vi "CANOpen_NMT_Main.vi"(6 "EM GB NG conf":T3(array[cluster])=[{"Emergency"={"Enable"=TRUE}, "Heartbeat and Node Guarding"={"Mode"=enum."None", "Guard Time (ms)"=5, "Consumer Time (ms)"=5}}, {"Emergency"={"Enable"=TRUE}, "Heartbeat and Node Guarding"={"Mode"=enum."None", "Guard Time (ms)"=5, "Consumer Time (ms)"=5}}], 7 "Period":i64=10, 8 "error in (no error)":errorcluster, 9 "stop in":bool, 10 "Nodes":T4[](array[typedef])=[{"RPDOs"=[], "TPDOs"=[], "Node ID"=1, "SDOs"=[], "Dynamic SDOs"=[], "NMT"={"Node run state"=0, "Emergency"=FALSE, "HB NG"={"Mode"=enum."NG", "Update Time"=128, "Static detect in None"=enum."HB"}, "Delay for opp. state (ms)"=5.0, "Node init static SDO state"=1, "Stop and Reset on Shutdown"=FALSE}}, {"RPDOs"=[], "TPDOs"=[], "Node ID"=2, "SDOs"=[], "Dynamic SDOs"=[], "NMT"={"Node run state"=0, "Emergency"=FALSE, "HB NG"={"Mode"=enum."NG", "Update Time"=128, "Static detect in None"=enum."HB"}, "Delay for opp. state (ms)"=5.0, "Node init static SDO state"=1, "Stop and Reset on Shutdown"=FALSE}}] {"NMT"."Node init static SDO state" items=["start remote node"=1, "enter pre-operational"=128]; "NMT"."Node run state" items=["start remote node"=1, "stop remote node"=2, "enter pre-operational"=128, "reset node"=129, "reset communication"=130]; "Dynamic SDOs"."Sub-Index (0)" format="%.0x"; "Dynamic SDOs"."Object Index" format="%.0x"; "Dynamic SDOs"."Block Data" format="%.0x"; "RPDOs"."PDO Channel" items=["PDO 1", "PDO 2", "PDO 3", "PDO 4"]; "RPDOs"."Parameters"."Bit Offset" max=8 step=1; "RPDOs"."Parameters"."Byte Offset" max=8 step=1; "TPDOs"."PDO Channel" items=["PDO 1", "PDO 2", "PDO 3", "PDO 4"]; "TPDOs"."Parameters"."Bit Offset" max=8 step=1; "TPDOs"."Parameters"."Byte Offset" max=8 step=1; "SDOs"."Sub-Index (0)" format="%.0x"; "SDOs"."Object Index" format="%.0x"; "SDOs"."Block Data" format="%.0x"}, 11 "interface object in":refnum<k20>) -> (0 "error out":errorcluster, 1 "Timestamp":timestamp, 2 "emergency message":T13 {"manufacturer specific error field" format="%.0x"; "error register" format="%.0x"; "error code" format="%.0x"}, 3 "interface object out":refnum<k20>, 5 "Is New?":bool)   [LabVIEW 2021, in "CANOpen Addon Engine.lvlib"]
uses:
  CANOpen Addon Engine.lvlib
  SubVIS/CANOpen_Node Message Settings.ctl
  Shared/CANOpen_PDO Settings.ctl
  Shared/CANOpen_PDO Parameter Settings.ctl
  Shared/CANOpen_PDO Data Type.ctl
  Shared/CANopen Byte Order.ctl
  Shared/CANOpen_SDO Settings.ctl
  SubVIS/CANOpen_NMT Settings.ctl
  Shared/CanOpen_NMT_Config.ctl
  Shared/CanOpen_NMT_Static detect.ctl
  Shared/CANOpen_Emergency Settings.ctl
  Shared/CANOpen_Heartbeat and Node Guarding Settings.ctl
  Emergency VI states.ctl
  <vilib>/Platform/TimedLoop/XDataNode/timing_clust.ctl
  <vilib>/Platform/TimedLoop/XDataNode/nitl_modes.ctl
  <vilib>/Platform/TimedLoop/XDataNode/wakeup.ctl
  <vilib>/CANopenLib/CANOPEN.llb/CANopen Emergency Create.vi
  <vilib>/CANopenLib/CANOPEN.llb/CANopen Emergency Start.vi
  <vilib>/CANopenLib/CANOPEN.llb/CANopen Emergency Read.vi
  <vilib>/CANopenLib/CANOPEN.llb/CANopen Emergency Close.vi
  <vilib>/Platform/TimedLoop/XDataNode/XDataNode.xnode
  <vilib>/Platform/TimedLoop/XDataNode/XDNodeRunTimeDep.lvlib
  Shared/CANOpen Addon Shared.lvlib
panel:
  # "LSB"
  # "MSB"
  # "LSB"
  # "MSB"
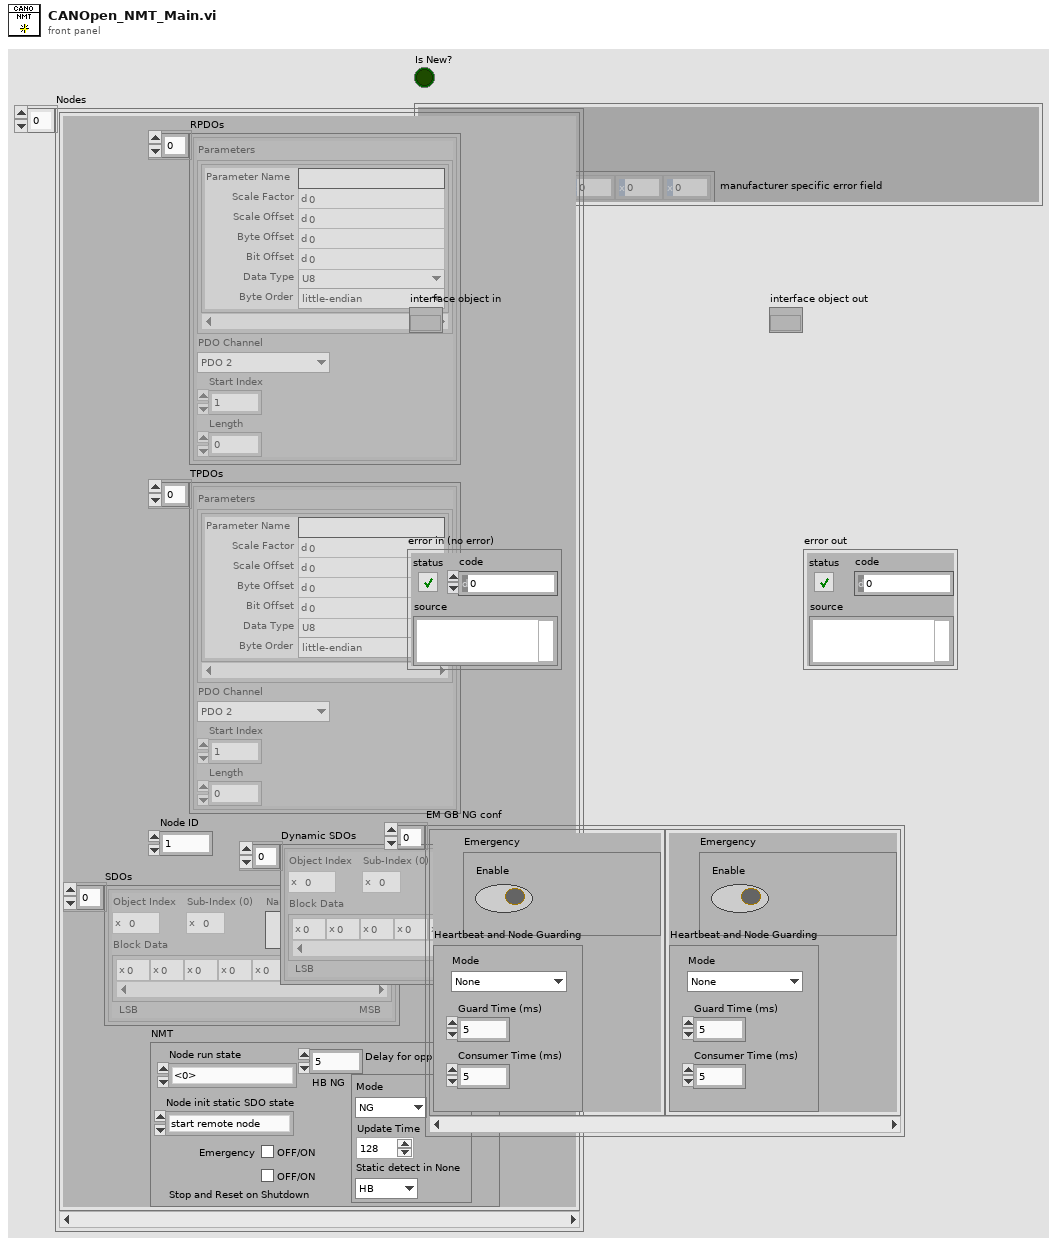
[diagram p1: front panel]
types:
  T1 = typedef "CANOpen Addon Shared.lvlib/CANOpen_Emergency Settings.ctl" = cluster{"Enable":bool}
  T2 = typedef "CANOpen Addon Shared.lvlib/CANOpen_Heartbeat and Node Guarding Settings.ctl" = cluster{"Mode":enum16{"None", "Hearbeat", "Node Guarding"}, "Guard Time (ms)":u16, "Consumer Time (ms)":u16}
  T3 = cluster{"Emergency":T1, "Heartbeat and Node Guarding":T2}[]
  T4 = typedef "CANOpen Addon Engine.lvlib/CANOpen_Node Message Settings.ctl" = cluster{"RPDOs":T5[], "TPDOs":T5[], "Node ID":u8, "SDOs":T9[], "Dynamic SDOs":T9[], "NMT":T10}
  T5 = typedef "CANOpen Addon Shared.lvlib/CANOpen_PDO Settings.ctl" = cluster{"Parameters":T6[], "PDO Channel":u8, "Start Index":u32, "Length":u32}
  T6 = typedef "CANOpen Addon Shared.lvlib/CANOpen_PDO Parameter Settings.ctl" = cluster{"Parameter Name":string, "Scale Factor":dbl, "Scale Offset":dbl, "Byte Offset":u8, "Bit Offset":u8, "Data Type":T7, "Byte Order":T8}
  T7 = typedef "CANOpen Addon Shared.lvlib/CANOpen_PDO Data Type.ctl" = enum16{"U8", "U16", "U32", "I8", "I16", "I32", "Single", "Double", "Boolean"}
  T8 = typedef "CANOpen Addon Shared.lvlib/CANopen Byte Order.ctl" = enum16{"big-endian network order", "little-endian"}
  T9 = typedef "CANOpen Addon Shared.lvlib/CANOpen_SDO Settings.ctl" = cluster{"Object Index":u16, "Sub-Index (0)":u8, "Block Data":u8[], "Name":string}
  T10 = typedef "CANOpen Addon Engine.lvlib/CANOpen_NMT Settings.ctl" = cluster{"Node run state":u16, "Emergency":bool, "HB NG":T11, "Delay for opp. state (ms)":dbl, "Node init static SDO state":u16, "Stop and Reset on Shutdown":bool}
  T11 = typedef "CANOpen Addon Shared.lvlib/CanOpen_NMT_Config.ctl" = cluster{"Mode":T12, "Update Time":u16, "Static detect in None":T12}
  T12 = typedef "CANOpen Addon Shared.lvlib/CanOpen_NMT_Static detect.ctl" = enum16{"None", "HB", "NG"}
  T13 = cluster{"error code":u16, "error register":u8, "manufacturer specific error field":u8[]}
  T14 = typedef "CANOpen Addon Engine.lvlib/Emergency VI states.ctl" = enum16{"Init", "Running ", "Shutdown"}
  T15 = typedef "XDNodeRunTimeDep.lvlib/timing_clust.ctl" = cluster{"Expected End [f-1]":u64, "Actual End [f-1]":u64, "Finished Late? [f-1]":bool, "Expected End [i-1]":u64, "Actual End [i-1]":u64, "Finished Late? [i-1]":bool, "Expected Start [i]":u64, "Actual Start [i]":u64, "Expected Start [f]":u64, "Actual Start [f]":u64, "Source Name":string, "Structure Name":string, "Period":i64, "Deadline":i64, "Offset":i64, "Start":i64, "Priority":i32, "Timeout":i32, "Mode":T16, "Wakeup Reason":T17, "Error":errorcluster, "Source Type":string, "Secondary Source Type":string, "Global End Time":u64, "Global Start Time":u64, "Frame Duration":u64, "Iteration Duration":u64, "Assigned CPU":i32, "I/O Scan Engine Mode":u32}
  T16 = typedef "XDNodeRunTimeDep.lvlib/nitl_modes.ctl" = enum32{"No Change", "Process missed periods, maintain original phase", "Discard missed periods, maintain original phase", "Process missed periods, ignore original phase", "Discard missed periods, ignore original phase"}
  T17 = typedef "XDNodeRunTimeDep.lvlib/wakeup.ctl" = enum32{"Normal", "Aborted", "Asynchronous wakeup", "Timing source error", "Timed loop error", "Timeout"}
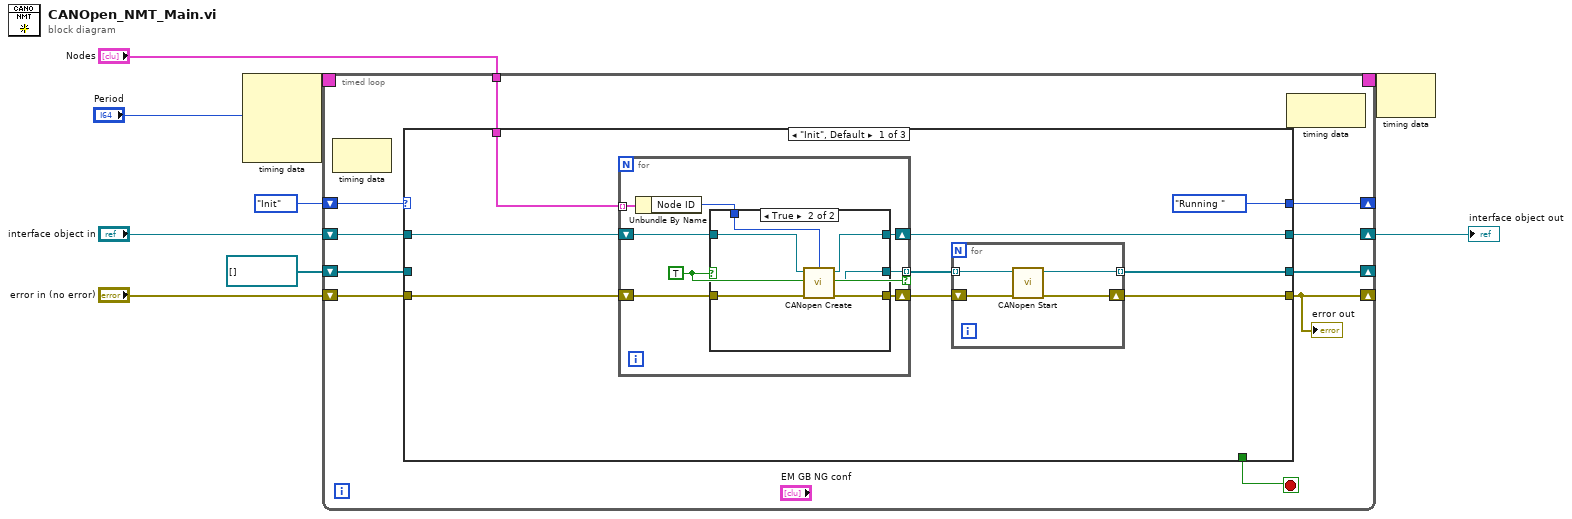
[diagram p0: block diagram]
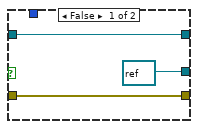
[diagram p2: hidden frame]
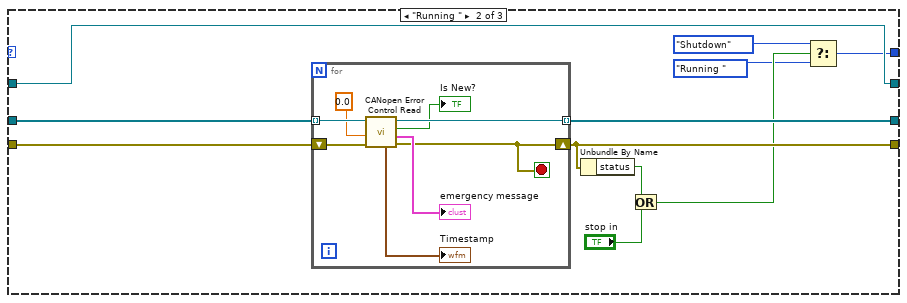
[diagram p3: hidden frame]
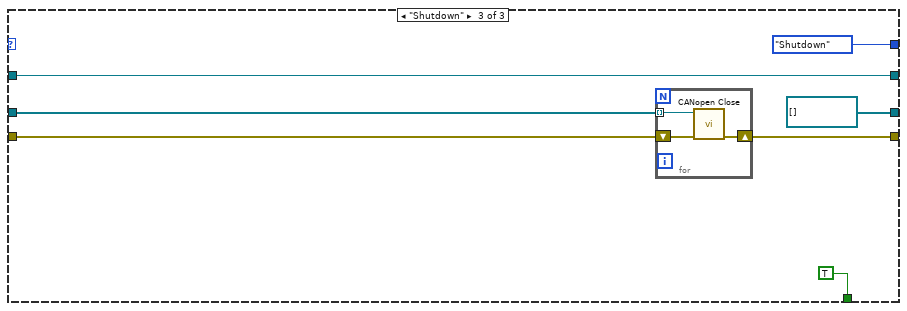
[diagram p4: hidden frame]
diagram:
  n1 = node-c288("Period") -> (w7:T15)  [unwired: 3 in]
  n2 = timed-loop {
    shift-right: [w18] -> _
    shift-left: Emergency_VI_states."Init" -> [w19]
    shift-right: [w13] -> _
    shift-left: refnum<k20>[] [] -> [w15]
    shift-right: [w11] -> _
    shift-left: "error in (no error)" -> [w16]
    shift-right: [w14] -> w5
    shift-left: "interface object in" -> [w12]
    timing: w7 -> [_]
    timing-out: [_] -> w6
    tunnel: "Nodes" -> [w10]
    stop <- w17 stop-if-true
    n3 = node-c288() -> ()  [unwired: 1 in, 1 out]
    n4 = case shown="\"Init\", Default" w19 {
      tunnel: [Emergency_VI_states."Running " w54 Emergency_VI_states."Shutdown"] -> w18
      tunnel: [_ _ TRUE] -> w17
      tunnel: w16 -> [w22 w57 w74]
      tunnel: [w28 w56 w73] -> w11
      tunnel: w15 -> [_ w62 w75]
      tunnel: [w27 w60 w76] -> w14
      tunnel: [w26 w61 refnum<k20>[] []] -> w13
      tunnel: w12 -> [w24 w60 w76]
      tunnel: w10 -> [w23 _ _]
      frame "Init", Default {
        n5 = for {
          tunnel: w23 -> [w40] mode=indexing
          shift-right: [w42] -> w29
          shift-left: w22 -> [w39]
          shift-right: [w37] -> w27
          shift-left: w24 -> [w41]
          tunnel: [w36] -> w25 mode=indexing if=w35
          w35 = TRUE
          n6 = Unbundle By Name(w40) -> ("Node ID"=w38:u8)
          n7 = case shown="True" w35 {
            tunnel: [w45 w51] -> w42
            tunnel: [refnum<k20> refnum ("emergency object out") w50] -> w36
            tunnel: w41 -> [w44 w49]
            tunnel: w39 -> [w45 w48]
            tunnel: w38 -> [_ w47]
            tunnel: [w44 w46] -> w37
            frame False {
            }
            frame True {
              n8 = call-poly <vilib>:"CANopen Create.vi"("node-ID"=w47, "error in (no error)"=w48, "interface object in"=w49) -> ("error out"=w51:errorcluster, "emergency object out"=w50:refnum<k20>, "interface object out"=w46:refnum<k20>)  [unwired: 6 in]
            }
          }
        }
        n9 = for {
          tunnel: w25 -> [w33] mode=indexing
          tunnel: [w31] -> w26 mode=indexing
          shift-right: [w32] -> w28
          shift-left: w29 -> [w34]
          n10 = call-poly <vilib>:"CANopen Start.vi"("error in (no error)"=w34, "emergency object in"=w33) -> ("error out"=w32:errorcluster, "emergency object out"=w31:refnum<k20>)  [unwired: 8 in]
        }
      }
      frame "Running " {
        n11 = for {
          tunnel: w62 -> [w69] mode=indexing
          tunnel: [w68] -> w61 mode=indexing
          shift-right: [w63] -> w56
          shift-left: w57 -> [w64]
          stop <- w63 stop-if-true
          n12 = call-poly <vilib>:"CANopen Error Control Read.vi"("error in (no error)"=w64, "timeout (0s)"=0.0 ("timeout(0)"), "emergency object in"=w69) -> ("error out"=w63:errorcluster, "emergency message"=→"emergency message":T13, "new message?"=→"Is New?":bool, "emergency object out"=w68:refnum<k20>, "timestamp"=→"Timestamp":timestamp)  [unwired: 4 in]
        }
        n13 = Unbundle By Name(w56) -> ("status"=w58:bool)
        n14 = Or(x=w58, y="stop in") -> (x .or. y?=w55:bool)
        n15 = Select(t=Emergency_VI_states."Shutdown", s=w55, f=Emergency_VI_states."Running ") -> (s? t:f=w54:T14)
      }
      frame "Shutdown" {
        n16 = for {
          shift-right: [w80] -> w73
          shift-left: w74 -> [w79]
          tunnel: w75 -> [w78] mode=indexing
          n17 = call-poly <vilib>:"CANopen Close.vi"("error in (no error)"=w79, "emergency object in"=w78) -> ("error out"=w80:errorcluster)  [unwired: 9 in]
        }
      }
    }
    "error out" <- w11
    n18 = node-c288() -> ()  [unwired: 1 in, 1 out]
  }
  "interface object out" <- w5
  n19 = node-c288(w6) -> ()  [unwired: 1 out]
